vi "LoadDataPointsToFpgaMemory.vi"(8 "error in (no error)":errorcluster, 9 "NumDataPoints":u32, 10 "Work Unit Data Points":csg[](array[numeric]), 11 "SETI_LV_FPGA in":refnum<class "SETI_LV_FPGA.lvclass">) -> (0 "error out":errorcluster, 1 "NumDataPoints":u32, 2 "Work Unit Data Points":csg[](array[numeric]), 3 "SETI_LV_FPGA out":refnum<class "SETI_LV_FPGA.lvclass">)   [LabVIEW 2015, in "SETI_LV_FPGA.lvclass"]
uses:
  SETI_LV_FPGA.lvclass
  SETI_LV_FPGA.lvclass/SETI_LV_FPGA.ctl
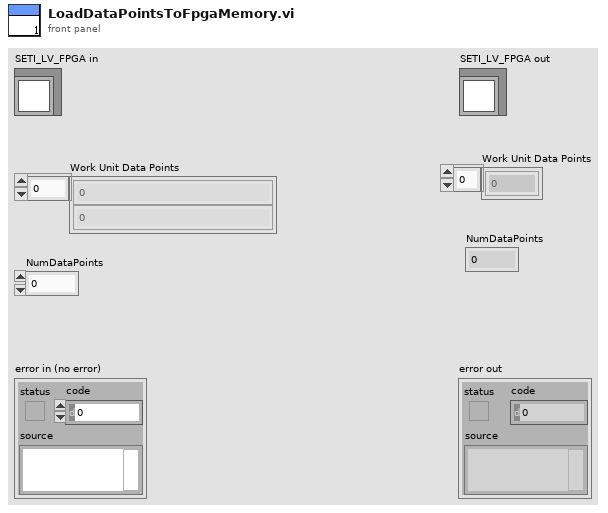
[diagram p1: front panel]
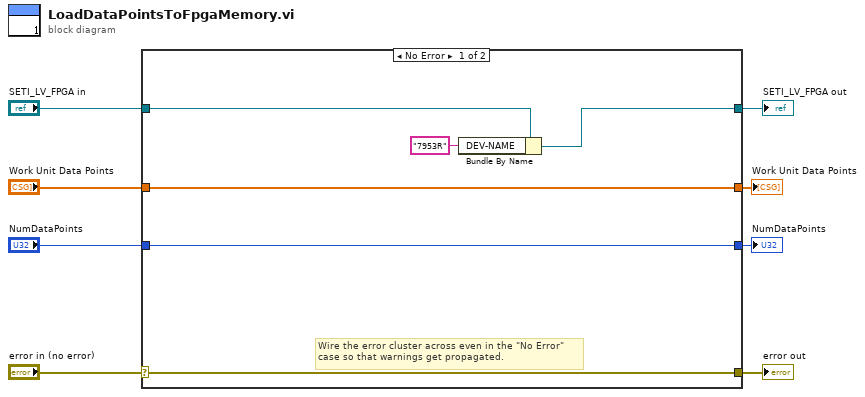
[diagram p0: block diagram]
diagram:
  n1 = case shown="No Error" "error in (no error)" {
    selector: "error in (no error)" -> [w14 w18]
    tunnel: [w14 w18] -> w7
    tunnel: [w13 w17] -> w5
    tunnel: "SETI_LV_FPGA in" -> [w12 w17]
    tunnel: [w10 w16] -> w1
    tunnel: "Work Unit Data Points" -> [w10 w16]
    tunnel: "NumDataPoints" -> [w9 w15]
    tunnel: [w9 w15] -> w2
    frame No Error {
      # "Wire the error cluster across even in the \"No Error\"\ncase so that warnings get propagated."
      n2 = Bundle By Name(cluster=w12, "DEV-NAME"="7953R") -> (w13:refnum<class "SETI_LV_FPGA.lvclass">)
    }
    frame Error {
    }
  }
  "error out" <- w7
  "SETI_LV_FPGA out" <- w5
  "NumDataPoints" <- w2
  "Work Unit Data Points" <- w1
